vi "SetJointRotation.vi"(8 "error in (no error)":errorcluster, 9 "Rotation (Deg)":dbl, 10 "JointType":enum16{"A_Shoulder", "B_Elbow", "C_Wrist"}(ring), 11 "Robot_Interface in":refnum<class "Robot_Interface.lvclass">) -> (0 "error out":errorcluster, 3 "Robot_Interface out":refnum<class "Robot_Interface.lvclass">)   [LabVIEW 2015, in "Robot_Interface.lvclass"]
uses:
  Robot_Interface.lvclass
  Robot_Interface.lvclass/Robot_Interface.ctl
  Subsytems/JKI.Robot.SMO.Base/JKI.Robot.SMO.Base.lvclass
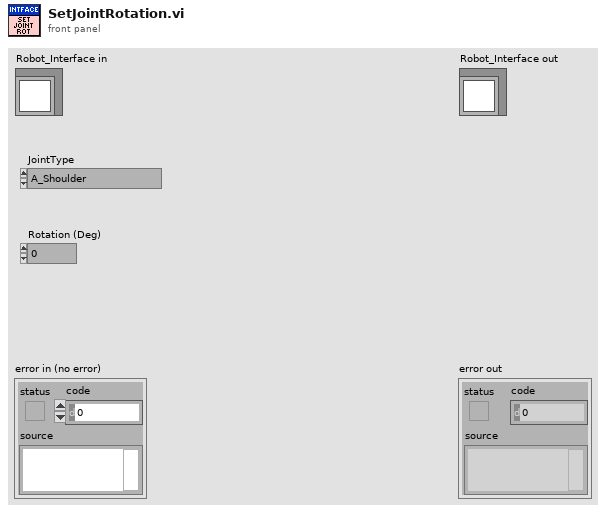
[diagram p1: front panel]
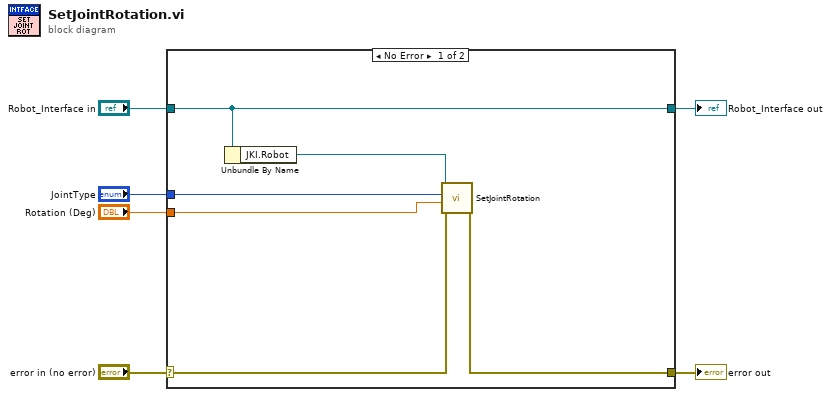
[diagram p0: block diagram]
diagram:
  n1 = case shown="No Error" "error in (no error)" {
    selector: "error in (no error)" -> [w12 w14]
    tunnel: [w11 w14] -> w5
    tunnel: [w8 w13] -> w3
    tunnel: "Robot_Interface in" -> [w8 w13]
    tunnel: "JointType" -> [w10 _]
    tunnel: "Rotation (Deg)" -> [w9 _]
    frame No Error {
      n2 = Unbundle By Name(w8) -> ("JKI.Robot"=w7:refnum<class "JKI.Robot.SMO.Base.lvclass">)
      n3 = call-dynamic "SetJointRotation.vi"("error in (no error)"=w12, "Rotation (Deg)"=w9, "Joint"=w10, "JKI.Robot.SMO.Base"=w7) -> ("error out"=w11:errorcluster)  [unwired: 6 in, 1 out]
    }
    frame Error {
    }
  }
  "error out" <- w5
  "Robot_Interface out" <- w3
